vi "Simulation.vi"(8 "error in (no error)":errorcluster, 11 "BattPack in":refnum<class "Battery Pack.lvclass">) -> (0 "error out":errorcluster)   [LabVIEW 2021, in "Battery Pack.lvclass"]
uses:
  Battery Pack.lvclass
  C:/S2L_Dev/LV2021/lv-Vessel_Simulator/MB Slave Simulator Base/MB Slave Simulator Base.lvclass
  C:/Program Files (x86)/National Instruments/LabVIEW 2021/user.lib/S2 Labs/Module Framework/Modules/Modbus/Modbus Slave Base/Modbus Slave Base.lvclass
  C:/Program Files (x86)/National Instruments/LabVIEW 2021/user.lib/S2 Labs/Module Framework/Modules/Base/Module.lvclass
  MB Slave Simulator Base/MB Slave Simulator Base.lvclass/MB Slave Simulator Base.ctl
  <userlib>/S2 Labs/Module Framework/Modules/Modbus/Modbus Slave Base/Modbus Slave Base.lvclass/Modbus Slave Base.ctl
  <userlib>/S2 Labs/CVT Toolkit/CVT.lvclass/CVT.ctl
  MB Slave Simulator Base/Accessors/Read Initialized.vi
  7fd4deaf-910a-4b91-88c3-86ab508fcff0.vi
  8b1d3db6-7cbb-494e-a33b-56b9f1ab6464.vi
  e29effdb-e71a-4654-a266-2ffe15539be1.vi
  <userlib>/S2 Labs/Module Framework/Modules/Modbus/Modbus Slave Base/Read MB Ref.vi
  8b1d3db6-7cbb-494e-a33b-56b9f1ab6464.vi/1553f4ce-967c-4f57-a913-5f155bf4374d.vi
  <userlib>/S2 Labs/CVT Toolkit/Read CVT DVR.vi
  Global.vi
  <userlib>/S2 Labs/Module Framework/Modules/Base/Get Module CVT Ref.vi
  <userlib>/S2 Labs/Modbus Toolkit/Slave/S2L Modbus Slave.lvclass
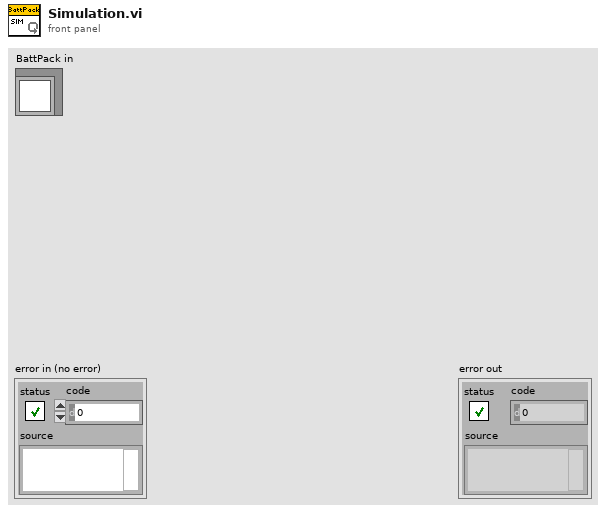
[diagram p1: front panel]
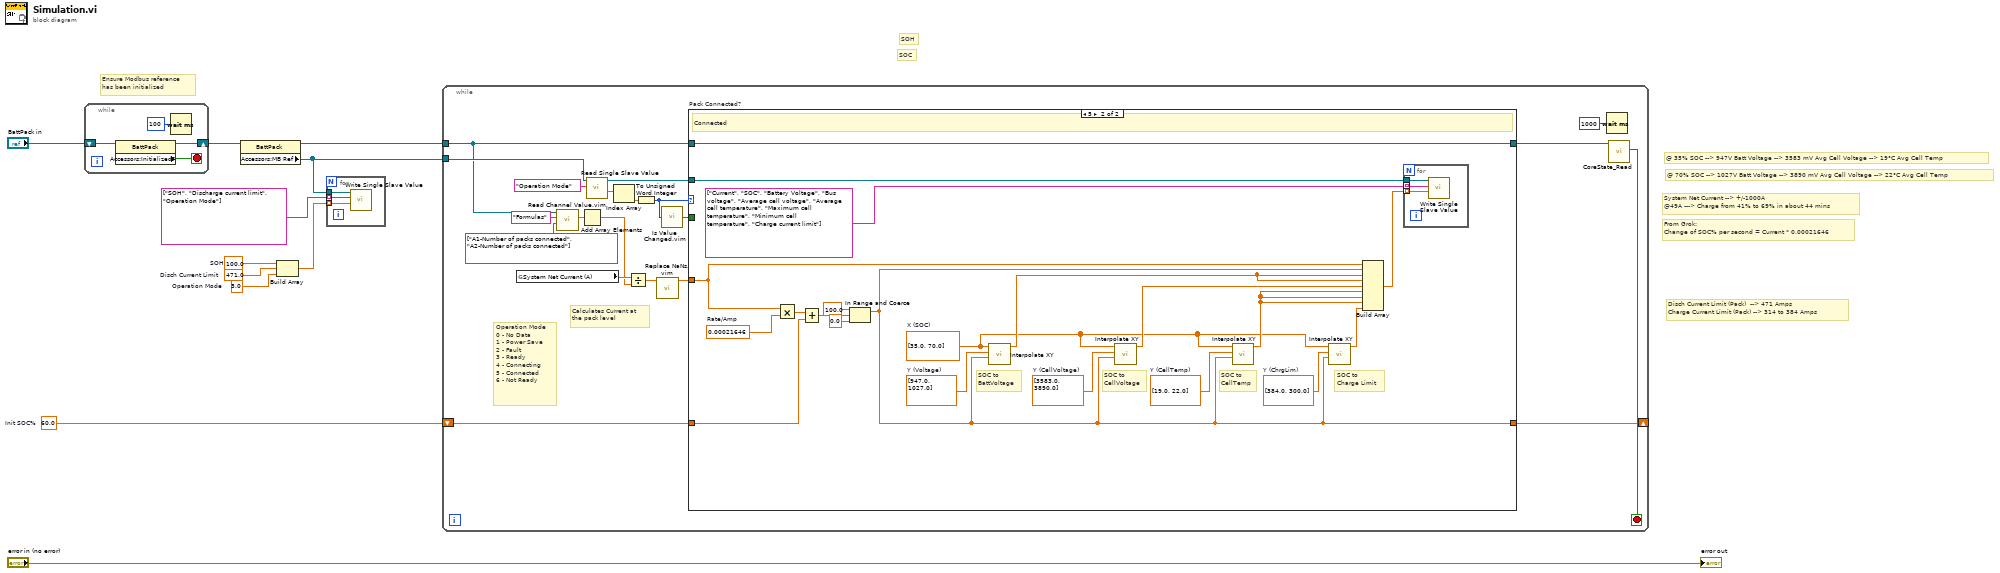
[diagram p0: block diagram]
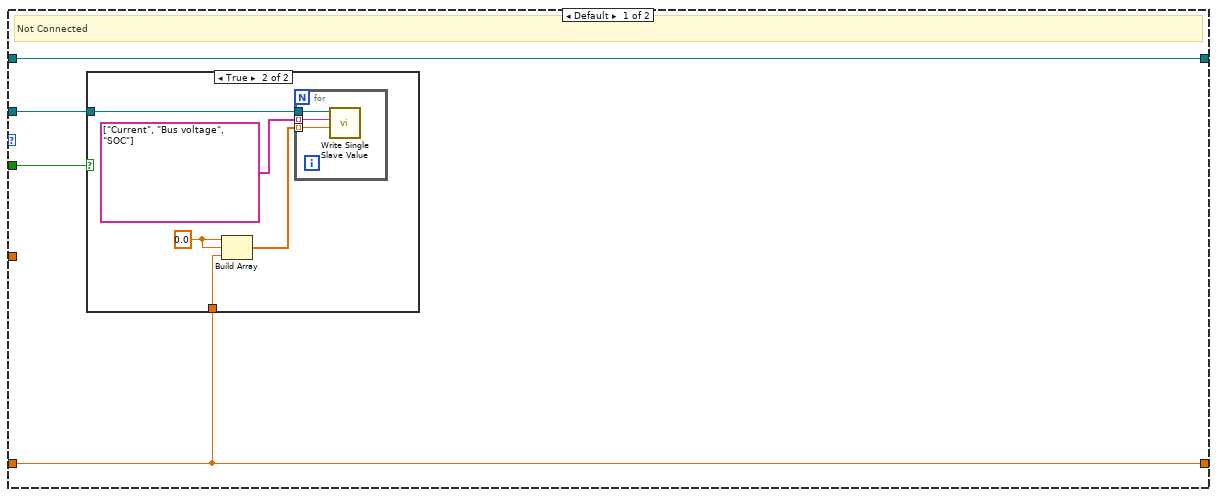
[diagram p2: hidden frame]
diagram:
  w2 = 3.0  # Operation Mode
  w3 = 471.0  # Disch Current Limit
  w4 = 100.0  # SOH
  w10 = 60.0  # Init SOC%
  # "Ensure Modbus reference\nhas been initialized"
  # "SOC"
  # "SOH"
  # "Disch Current Limit (Pack)  --> 471 Amps\nCharge Current Limit (Pack) --> 314 to 384 Amps"
  # "From Grok:\nChange of SOC% per second = Current * 0.00021646"
  # "System Net Current --> +/-1000A\n@49A ---> Charge from 41% to 69% in about 44 mins"
  # "@ 35% SOC --> 947V Batt Voltage --> 3583 mV Avg Cell Voltage --> 19°C Avg Cell Temp"
  # "@ 70% SOC --> 1027V Batt Voltage --> 3890 mV Avg Cell Voltage --> 22°C Avg Cell Temp"
  n1 = while {
    shift-right: [w13] -> w7
    shift-left: "BattPack in" -> [w14]
    stop <- w12 stop-if-true
    n2 = property class="BattPack"(reference=w14) -> (reference out=w13:refnum<class "Battery Pack.lvclass">, "Accessors:Initialized?"=w12:bool)  [unwired: 1 in, 1 out]
    n3 = Wait (ms)(milliseconds to wait=u32 100) -> ()  [unwired: 1 out]
  }
  n4 = property class="BattPack"(reference=w7) -> (reference out=w8:refnum<class "Battery Pack.lvclass">, "Accessors:MB Ref"=w6:refnum<class "S2L Modbus Slave.lvclass">)  [unwired: 1 in, 1 out]
  n5 = Build Array(w4, w3, w2) -> (w1:dbl[])
  n6 = for {
    tunnel: w6 -> [w18]
    tunnel: string[] ["SOH", "Discharge current limit", "Operation Mode"] ("Label") -> [w17] mode=indexing
    tunnel: w1 -> [w16] mode=indexing
    n7 = call-dynamic "Write Single Slave Value.vi"("Value"=w16, "Label"=w17, "S2L Modbus Slave in"=w18) -> ()  [unwired: 7 in, 2 out]
  }
  n8 = while {
    tunnel: w8 -> [w19]
    shift-right: [w30] -> _
    shift-left: w10 -> [w32]
    tunnel: w6 -> [w20]
    stop <- w38 stop-if-true
    # "Calculates Current at\nthe pack level"
    # "Operation Mode\n0 - No Data\n1 - Power Save\n2 - Fault\n3 - Ready\n4 - Connecting\n5 - Connected\n6 - Not Ready"
    n9 = global read "Global.vi" "System Net Current (A)"() -> (w26:dbl)
    n10 = call "Read Channel Value.vim"("Channel Label(s)"=string[] ["A1-Number of packs connected", "A2-Number of packs connected"] ("Label"), "Module"="Formulas", "Module in"=w19) -> ("value"=w27:dbl[])  [unwired: 2 in, 6 out]
    n11 = Add Array Elements(numeric array=w27) -> (sum=w25:dbl)
    n12 = call-dynamic "Read Single Slave Value.vi"("Label"="Operation Mode", "S2L Modbus Slave in"=w20) -> ("Value (s)"=w35:dbl[], "S2L Modbus Slave out"=w31:refnum<class "S2L Modbus Slave.lvclass">)  [unwired: 4 in, 4 out]
    n13 = Index Array(array=w35) -> (element=w34:dbl)  [unwired: 1 in]
    n14 = Divide(x=w26, y=w25) -> (x/y=w24:dbl)
    n15 = To Unsigned Word Integer(number=w34) -> (unsigned 16bit integer=w22:u16)
    n16 = call "Replace NaNs.vim"("Value In"=w24) -> ("Value Out"=w23:dbl)  [unwired: 9 in]
    n17 = call "Is Value Changed.vim"("value"=w22) -> ("changed or first call?"=w21:bool)
    n18 = case "Pack Connected?" shown="5" w22 {
      tunnel: [w42 w71] -> w33
      tunnel: w19 -> [w42 w71]
      tunnel: w32 -> [w39 w64]
      tunnel: w31 -> [w41 w70]
      tunnel: [w39 w53] -> w30
      tunnel: w23 -> [_ w67]
      tunnel: w21 -> [w40 _]
      frame Default {
        # "Not Connected"
        n19 = case shown="True" w40 {
          tunnel: w41 -> [_ w46]
          tunnel: w39 -> [_ w43]
          frame False {
          }
          frame True {
            w44 = 0.0
            n20 = Build Array(w44, w44, w43) -> (w45:dbl[])
            n21 = for {
              tunnel: w46 -> [w50]
              tunnel: string[] ["Current", "Bus voltage", "SOC"] ("Label") -> [w49] mode=indexing
              tunnel: w45 -> [w48] mode=indexing
              n22 = call-dynamic "Write Single Slave Value.vi"("Value"=w48, "Label"=w49, "S2L Modbus Slave in"=w50) -> ()  [unwired: 7 in, 2 out]
            }
          }
        }
      }
      frame 5 {
        w52 = dbl[] [384.0, 300.0]  # Y (ChrgLim)
        w58 = dbl[] [19.0, 22.0]  # Y (CellTemp)
        w59 = dbl[] [3583.0, 3890.0]  # Y (CellVoltage)
        w60 = dbl[] [947.0, 1027.0]  # Y (Voltage)
        w54 = dbl[] [35.0, 70.0]  # X (SOC)
        w66 = 0.00021646  # Rate/Amp
        # "SOC to \nCharge Limit"
        # "SOC to \nCellTemp"
        # "SOC to \nCellVoltage"
        # "SOC to \nBattVoltage"
        # "Connected"
        n23 = Multiply(x=w67, y=w66) -> (x*y=w65:dbl)
        n24 = Add(x=w65, y=w64) -> (x+y=w63:dbl)
        n25 = In Range and Coerce(upper limit=100.0, x=w63, lower limit=0.0) -> (coerced(x)=w53:dbl)  [unwired: 1 out]
        n26 = call <userlib>:"Interpolate XY.vi"("New X Value"=w53, "Y Values"=w60, "X Values"=w54) -> ("Y Value"=w56:dbl)  [unwired: 8 in]
        n27 = call <userlib>:"Interpolate XY.vi"("New X Value"=w53, "Y Values"=w59, "X Values"=w54) -> ("Y Value"=w57:dbl)  [unwired: 8 in]
        n28 = call <userlib>:"Interpolate XY.vi"("New X Value"=w53, "Y Values"=w58, "X Values"=w54) -> ("Y Value"=w55:dbl)  [unwired: 8 in]
        n29 = call <userlib>:"Interpolate XY.vi"("New X Value"=w53, "Y Values"=w52, "X Values"=w54) -> ("Y Value"=w51:dbl)  [unwired: 8 in]
        n30 = Build Array(w67, w53, w56, w56, w57, w55, w55, w55, w51) -> (w68:dbl[])
        n31 = for {
          tunnel: w70 -> [w74]
          tunnel: string[] ["Current", "SOC", "Battery Voltage", "Bus voltage", "Average cell voltage", "Average cell temperature", "Maximum cell temperature", "Minimum cell temperature", "Charge current limit"] ("Label") -> [w73] mode=indexing
          tunnel: w68 -> [w72] mode=indexing
          n32 = call-dynamic "Write Single Slave Value.vi"("Value"=w72, "Label"=w73, "S2L Modbus Slave in"=w74) -> ()  [unwired: 7 in, 2 out]
        }
      }
    }
    n33 = Wait (ms)(milliseconds to wait=u32 1000) -> ()  [unwired: 1 out]
    n34 = call-dynamic "CoreState_Read.vi"("Module in"=w33) -> ("Stopped?"=w38:bool)  [unwired: 8 in, 2 out]
  }
  "error out" <- "error in (no error)"
